vi "SeCrTs-RT_Global_R.vi"() -> ()   [LabVIEW 2022 SP3]
uses:
  RT Controls/SeCrTs-Message Cluster_R.ctl
  RT Controls/SeCrTs-Data Type Control screen.ctl
panel:
  in  "RT Writer Stream_DD":refnum<k21>
  in  "RT Writer Stream_D":refnum<k21>
  in  "RT Writer Stream_C":refnum<k21>
  in  "RT Stream Name_D":string="Command Stream from RT"
  in  "RT Stream Name_DD":string="Command Stream from RT"
  in  "Lconnection ID":refnum<k5>
  in  "Aconnection ID":refnum<k5>
  out "DriveL_Enable":bool
  out "DriveA_Enable":bool
  in  "UI Writer stream":refnum<k21>
  in  "UI Stream Name":string="/command/Target"
  in  "RT Stream Name_C":string="/data/writer"
  in  "Network Stream Polling Timeout (ms)":i32=10
  in  "Network Stream Connect Timeout (ms)":i32=-1
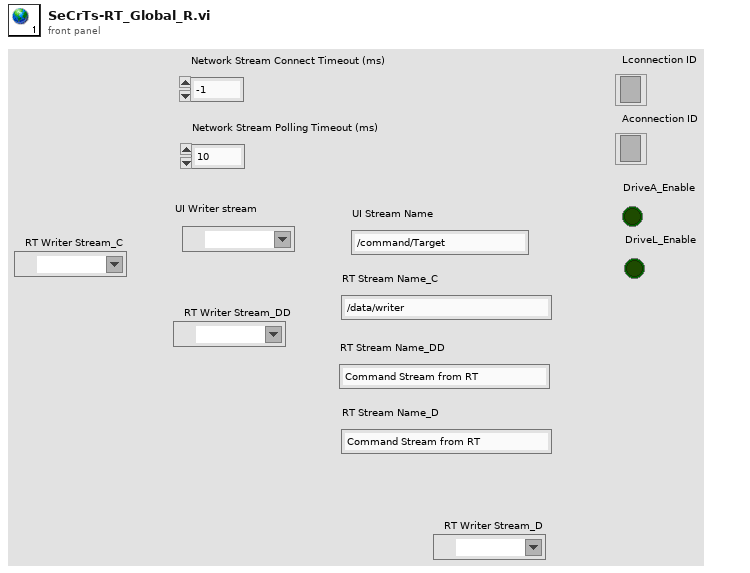
[diagram p1: front panel]
diagram:
